vi "FRCts20_Backend_DateString_to_TimeStamp.vi"(11 "DateTime String":string) -> (3 "Time Stamp":timestamp=timestamp(3403656258 s since 1904-01-01))   [LabVIEW 2014, in "FRCts20_Backend_Engine.lvlib"]
uses:
  FRCts20_Backend_Engine.lvlib
  <vilib>/Utility/miscctls.llb/LVDateTimeRec.ctl
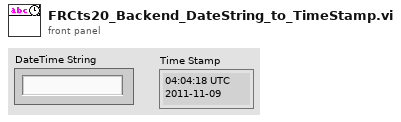
[diagram p1: front panel]
types:
  T1 = typedef "LVDateTimeRec.ctl" = cluster{"fractional second":dbl, "second":i32, "minute":i32, "hour":i32, "day of month":i32, "month":i32, "year":i32, "day of week":i32, "day of year":i32, "DST":i32}
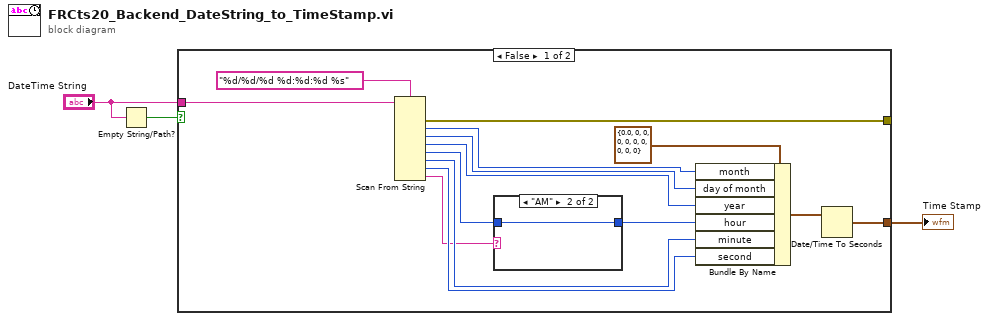
[diagram p0: block diagram]
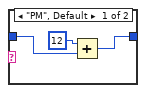
[diagram p2: hidden frame]
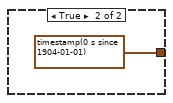
[diagram p3: hidden frame]
diagram:
  n1 = Empty String/Path?(string/path="DateTime String") -> (empty?=w3:bool)
  n2 = case shown="False" w3 {
    tunnel: [w7 timestamp(0 s since 1904-01-01)] -> w2
    tunnel: "DateTime String" -> [w17 _]
    tunnel: [w15 _] -> _
    frame False {
      n3 = Scan From String(format string="%d/%d/%d %d:%d:%d %s", input string=w17) -> (error out=w15:errorcluster, output 1=w13:i32, output 2=w12:i32, output 3=w11:i32, output 4=w5:i32, output 5=w10:i32, output 6=w9:i32, output 7=w6:string)  [unwired: 9 in, 2 out]
      n4 = case shown="\"AM\"" w6 {
        tunnel: w5 -> [w20 w21]
        tunnel: [w18 w21] -> w4
        frame "PM", Default {
          n5 = Add(x=12, y=w20) -> (x+y=w18:i32)
        }
        frame "AM" {
        }
      }
      n6 = Bundle By Name(cluster=T1 {"fractional second"=0.0, "second"=0, "minute"=0, "hour"=0, "day of month"=0, "month"=0, "year"=0, "day of week"=0, "day of year"=0, "DST"=0} ("date time rec"), "month"=w13, "day of month"=w12, "year"=w11, "hour"=w4, "minute"=w10, "second"=w9) -> (w8:T1)
      n7 = Date/Time To Seconds(2:w8) -> (0:w7:timestamp)  [unwired: 1 in]
    }
    frame True {
    }
  }
  "Time Stamp" <- w2
